vi "To and From Array Test.vi"() -> (0 "error out":errorcluster, 2 "Pass":bool)   [LabVIEW 2017, in "J1939 tests.lvlib"]
uses:
  J1939 tests.lvlib
  module/configuration/J1939 configuration.lvclass/J1939 configuration.ctl
  <vilib>/NI/Tag Bus Module Framework/channel/TBM channel.lvclass
  module/configuration/J1939 configuration.lvclass
panel:
  out "Class Equal":bool
  out "Lines Equal":bool
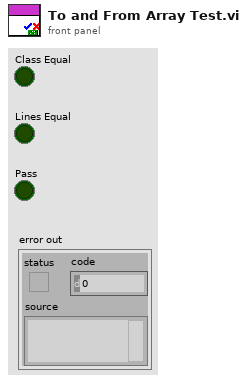
[diagram p1: front panel]
types:
  T1 = typedef "J1939 configuration.lvclass/Line.ctl" = cluster{"channel":refnum<class "TBM channel.lvclass">, "XNET Signal":refnum<k21>}
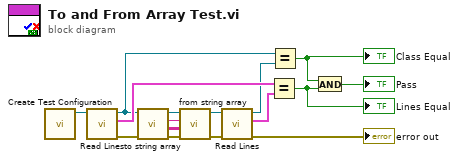
[diagram p0: block diagram]
diagram:
  n1 = call "Create Test Configuration.vi"() -> ("Module Configuration"=w16:refnum<class "J1939 configuration.lvclass">)  [unwired: 5 in, 6 out]
  n2 = call "Read Lines.vi"("J1939 configuration in"=w16) -> ("error out"=w12:errorcluster, "Lines"=w9:T1[], "J1939 configuration out"=w5:refnum<class "J1939 configuration.lvclass">)  [unwired: 8 in]
  n3 = call-dynamic "to string array.vi"("error in (no error)"=w12, "module configuration in"=w5) -> ("error out"=w13:errorcluster, "Array"=w14:string[][], "version"=w15:string, "module configuration out"=w10:refnum<class "J1939 configuration.lvclass">)  [unwired: 6 in]
  n4 = call-dynamic "from string array.vi"("error in (no error)"=w13, "String Array"=w14, "version"=w15, "module configuration in"=w10) -> ("error out"=w11:errorcluster, "module configuration out"=w7:refnum<class "J1939 configuration.lvclass">)  [unwired: 6 in]
  n5 = call "Read Lines.vi"("error in (no error)"=w11, "J1939 configuration in"=w7) -> ("error out"=→"error out":errorcluster, "Lines"=w8:T1[], "J1939 configuration out"=w6:refnum<class "J1939 configuration.lvclass">)  [unwired: 7 in]
  n6 = Equal?(x=w9, y=w8) -> (x = y?=w3:bool)
  "Lines Equal" <- w3
  n7 = Equal?(x=w5, y=w6) -> (x = y?=w4:bool)
  "Class Equal" <- w4
  n8 = And(x=w4, y=w3) -> (x .and. y?=→"Pass":bool)
